vi "Actor Core.vi"(8 "error in":errorcluster, 11 "Sim GPS in":refnum<class "Sim GPS.lvclass">) -> (0 "error out":errorcluster, 3 "Actor out":refnum<class "Actor.lvclass">)   [LabVIEW 2015, in "Sim GPS.lvlib" / "Sim GPS.lvclass"]
doc: "(<B>Filename</B>: Actor Framework.lvlib:Actor.lvclass:Actor Core.vi)\n\nReceives messages to the actor, reacts to them, and initiates any error handling that may shut the actor down.\n\nDescendant classes may override this VI to append parallel tasks for the actor to complete while it handles messages. Overrides use the Call Parent Method node."
uses:
  Sim GPS.lvclass
  Actors/RDS Parent Actor/RDS Parent Actor/RDS Parent Actor.lvclass
  Libraries/RDS Framework/RDS Message ID.ctl
  Libraries/RDS Child Messages/RDS Child Messages.lvlib
  Libraries/RDS Framework/RDS Message Class/RDS Message.lvclass
  <vilib>/ActorFramework/Actor/Actor.lvclass
  Libraries/RDS Child Messages/GPS Data Message/GPS Data Message.lvclass
  Libraries/3rd Party/NMEA_GPS/NMEA_LatitudeDirection.ctl
  Libraries/3rd Party/NMEA_GPS/NMEA.lvlib
  Libraries/3rd Party/NMEA_GPS/NMEA_LongitudeDirection.ctl
  Libraries/3rd Party/NMEA_GPS/NMEA_GPRMC-data.ctl
panel:
  in  "GPRMC-data":T1={"TimeStamp"=timestamp(0 s since 1904-01-01), "Validity"=FALSE, "Latitude"=0.0, "Latitude-Direction"=enum."North", "Longitude"=0.0, "Longitude-Direction"=enum."East", "Speed in knots"=0.0, "True course"=0.0, "Date Stamp"=timestamp(0 s since 1904-01-01), "Magnetic Variation (East/West)"=0.0, "GPS Latitude"=0.0, "GPS Longitude"=0.0} {"GPS Longitude" format="%.6f"; "GPS Latitude" format="%.6f"; "Magnetic Variation (East/West)" format="%.02f [deg]"; "Date Stamp" format="%<%x>T"; "True course" format="%.02f [deg]"; "Speed in knots" format="%.02f [kts]"; "Longitude" format="%0.4f [long]"; "Latitude" format="%.04f [lat]"; "TimeStamp" format="%<%.2X>T"}
  in  "OK Button":bool
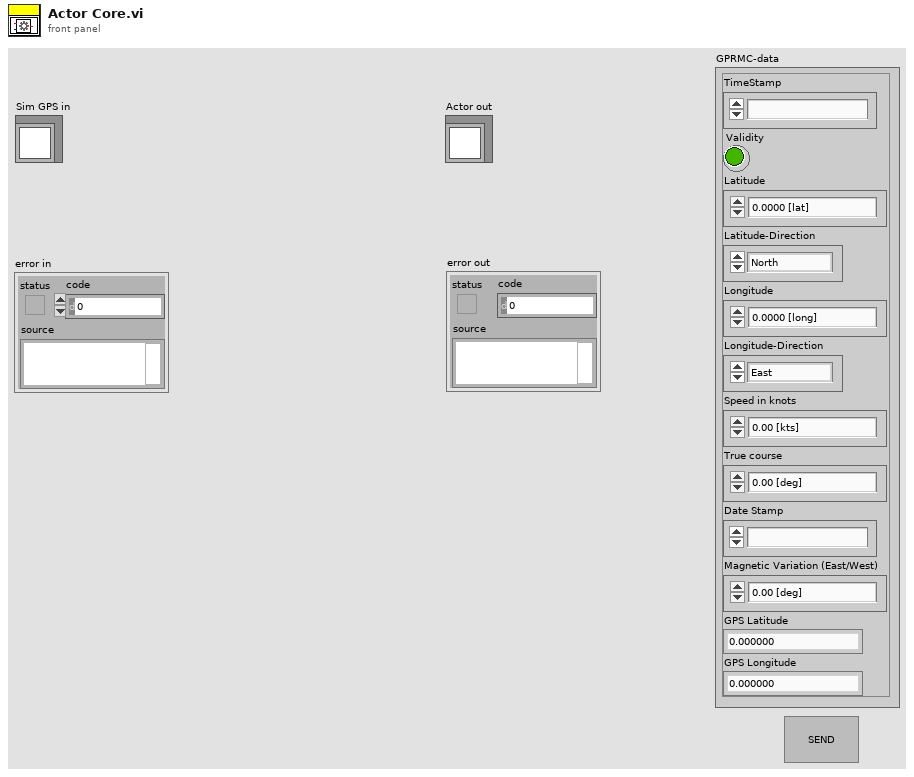
[diagram p1: front panel]
types:
  T1 = typedef "RDS Libraries.lvlib/NMEA.lvlib/NMEA_GPRMC-data.ctl" = cluster{"TimeStamp":timestamp, "Validity":bool, "Latitude":dbl, "Latitude-Direction":T2, "Longitude":dbl, "Longitude-Direction":T3, "Speed in knots":sgl, "True course":sgl, "Date Stamp":timestamp, "Magnetic Variation (East/West)":sgl, "GPS Latitude":dbl, "GPS Longitude":dbl}
  T2 = typedef "RDS Libraries.lvlib/NMEA.lvlib/NMEA_LatitudeDirection.ctl" = enum16{"", "North", "South"}
  T3 = typedef "RDS Libraries.lvlib/NMEA.lvlib/NMEA_LongitudeDirection.ctl" = enum16{"", "East", "West"}
  T4 = typedef "RDS Child Messages.lvlib/RDS Message ID.ctl" = enum16{"RDS Hello World", "String Message", "AIP_Status", "AIP_Command", "GPS_Data", "MCB_Command", "MCB_Status", "Compass_Data", "Depth_Data", "Battery_Data", "Contoller_State", "Set_Mag_Dev", "BTB_Shutdown", "State_Sample_Request", "State_Sample", "PID_Gains_Set", "Helm_Limiter_Set", "Helm_Heading_Command", "Helm_Steering_Command", "Helm_Status", "Controller_Message", "AIP_Set_Min_Depth", "Mission_Controller_State", "Mission_Upload", "Mission_Set_Op_and_Run", "Mission_Settings_Set"}
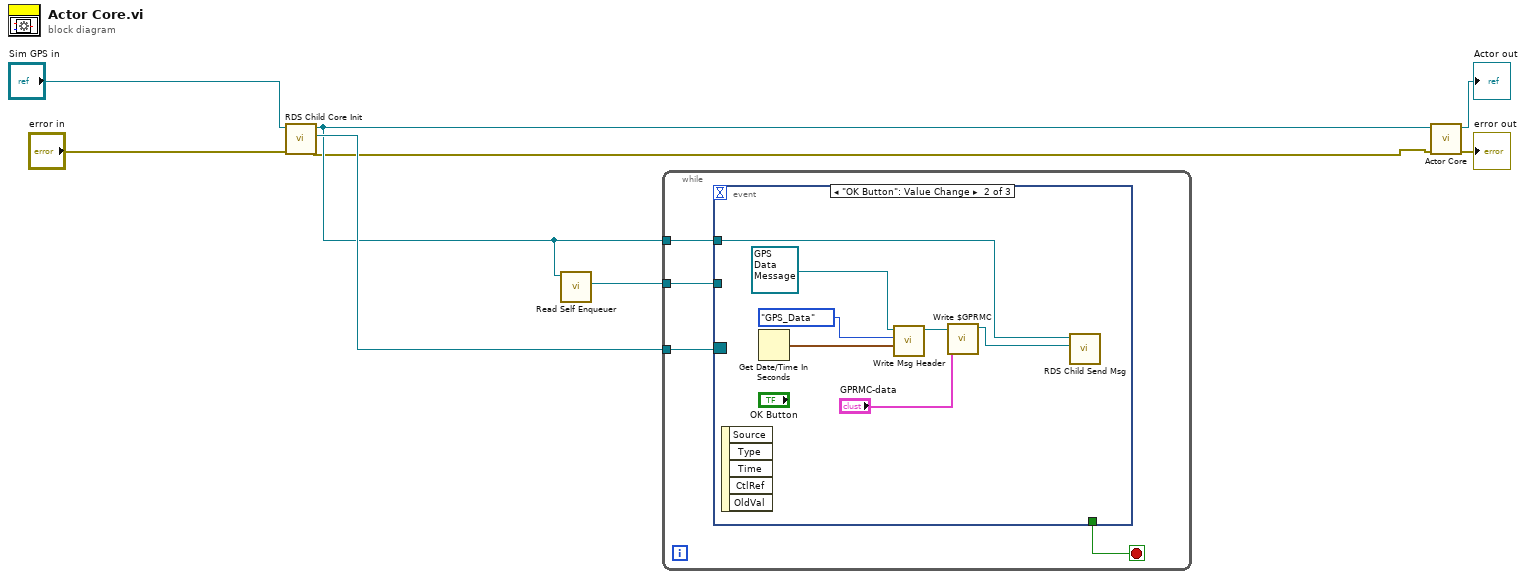
[diagram p0: block diagram]
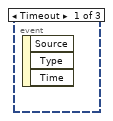
[diagram p2: hidden frame]
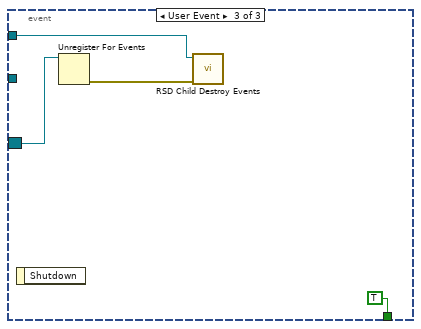
[diagram p3: hidden frame]
diagram:
  n1 = call "RDS Child Core Init.vi"("error in (no error)"="error in", "RDS Parent Actor in"="Sim GPS in") -> ("error out"=w3:errorcluster, "Event Registration Refnum"=w6:refnum<event-registration>, "RDS Parent Actor out"=w4:refnum<class "Sim GPS.lvclass">)  [unwired: 6 in, 1 out]
  n2 = call <vilib>:"Read Self Enqueuer.vi"("Actor"=w4) -> ("Self Enqueuer"=w5:refnum<class "Message Enqueuer.lvclass">)  [unwired: 10 in]
  n3 = while {
    tunnel: w6 -> [w11]
    tunnel: w4 -> [w12]
    tunnel: w5 -> [w9]
    stop <- w10 stop-if-true
    n4 = event shown="[1] \"OK Button\": Value Change" {
      selector: w11 -> [_ _ w21]
      dyn-events: _ -> [_ _ _]
      timeout: _ -> [_ _ _]
      tunnel: w12 -> [_ w17 w20]
      tunnel: [_ _ TRUE] -> w10
      tunnel: w9 -> [_ _ _]
      event Timeout {
        n5 = event-data() -> ()  [unwired: 1 in, 3 out]
      }
      event "OK Button": Value Change {
        n6 = event-data() -> ()  [unwired: 1 in, 5 out]
        n7 = Get Date/Time In Seconds() -> (seconds since 1Jan1904=w19:timestamp)
        n8 = call "Write Msg Header.vi"("Time Stamp"=w19, "Msg ID"=RDS_Message_ID."GPS_Data", "RDS Message in"=refnum<class "GPS Data Message.lvclass"> refnum ("RDS Child Messages.lvlib:GPS Data Message.lvclass")) -> ("RDS Message out"=w15:refnum<class "GPS Data Message.lvclass">)  [unwired: 7 in, 1 out]
        n9 = call "Write $GPRMC.vi"("GPRMC-data"="GPRMC-data", "GPS Data Message in"=w15) -> ("GPS Data Message out"=w13:refnum<class "GPS Data Message.lvclass">)  [unwired: 8 in, 1 out]
        n10 = call "RDS Child Send Msg.vi"("RDS Message"=w13, "RDS Parent Actor in"=w17) -> ()  [unwired: 8 in, 2 out]
      }
      event User Event {
        n11 = event-data() -> ()  [unwired: 1 in, 1 out]
        n12 = Unregister For Events(event registration refnum=w21) -> (error out=w22:errorcluster)  [unwired: 1 in]
        n13 = call "RSD Child Destroy Events.vi"("error in (no error)"=w22, "RDS Parent Actor in"=w20) -> ()  [unwired: 8 in, 2 out]
      }
    }
  }
  n14 = call-parent "Actor Core.vi"("error in"=w3, "Actor in"=w4) -> ("error out"=→"error out":errorcluster, "Actor out"=→"Actor out":refnum<class "Actor.lvclass">)  [unwired: 8 in]
